vi "Init.vi"(7 "Obj Dict":refnum<class "Object Dictionary.lvclass">, 8 "error in":errorcluster, 10 "Obj Entry":refnum<class "Object Entry.lvclass">, 11 "TPDO Mapping in":refnum<class "TPDO Mapping.lvclass">) -> (0 "error out":errorcluster, 3 "TPDO Mapping out":refnum<class "TPDO Mapping.lvclass">)   [LabVIEW 2020, in "CANopen.lvlib" / "TPDO Mapping.lvclass"]
uses:
  TPDO Mapping.lvclass
  Object Entry/Object Entry.lvclass
  Object Dictionary/Object Dictionary.lvclass
  PDO Mapping/PDO Mapping.lvclass
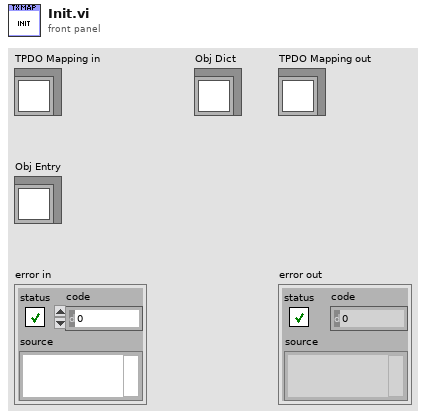
[diagram p1: front panel]
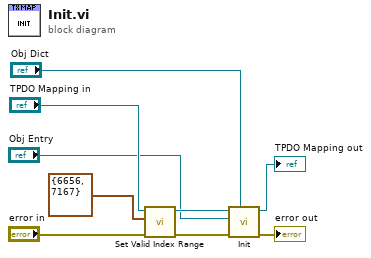
[diagram p0: block diagram]
diagram:
  n1 = call "Set Valid Index Range.vi"("error in"="error in", "Valid Index Range"=cluster{"Lower":u16, "Upper":u16} {"Lower"=6656, "Upper"=7167}, "PDO Mapping in"="TPDO Mapping in") -> ("error out"=w5:errorcluster, "PDO Mapping out"=w2:refnum<class "TPDO Mapping.lvclass">)  [unwired: 7 in]
  n2 = call-parent "Init.vi"("Obj Dict"="Obj Dict", "error in"=w5, "OD Entry"="Obj Entry", "PDO Mapping in"=w2) -> ("error out"=→"error out":errorcluster, "PDO Mapping out"=→"TPDO Mapping out":refnum<class "TPDO Mapping.lvclass">)  [unwired: 6 in]
